vi "inter cycle delay tester.vi"() -> ()   [LabVIEW 2021]
uses:
  <vilib>/Analysis/1siggen.llb/Ramp Pattern by Samples.vi
  <vilib>/Analysis/NI_AALBase.lvlib
panel:
  out "second subarray":bool[](array[boolean])
  out "unsigned 8bit integer":u8
  out "Waveform Graph":i16[][](graph)
  out "delayed data":i16[][](array[numeric])
  in  "delay":u8
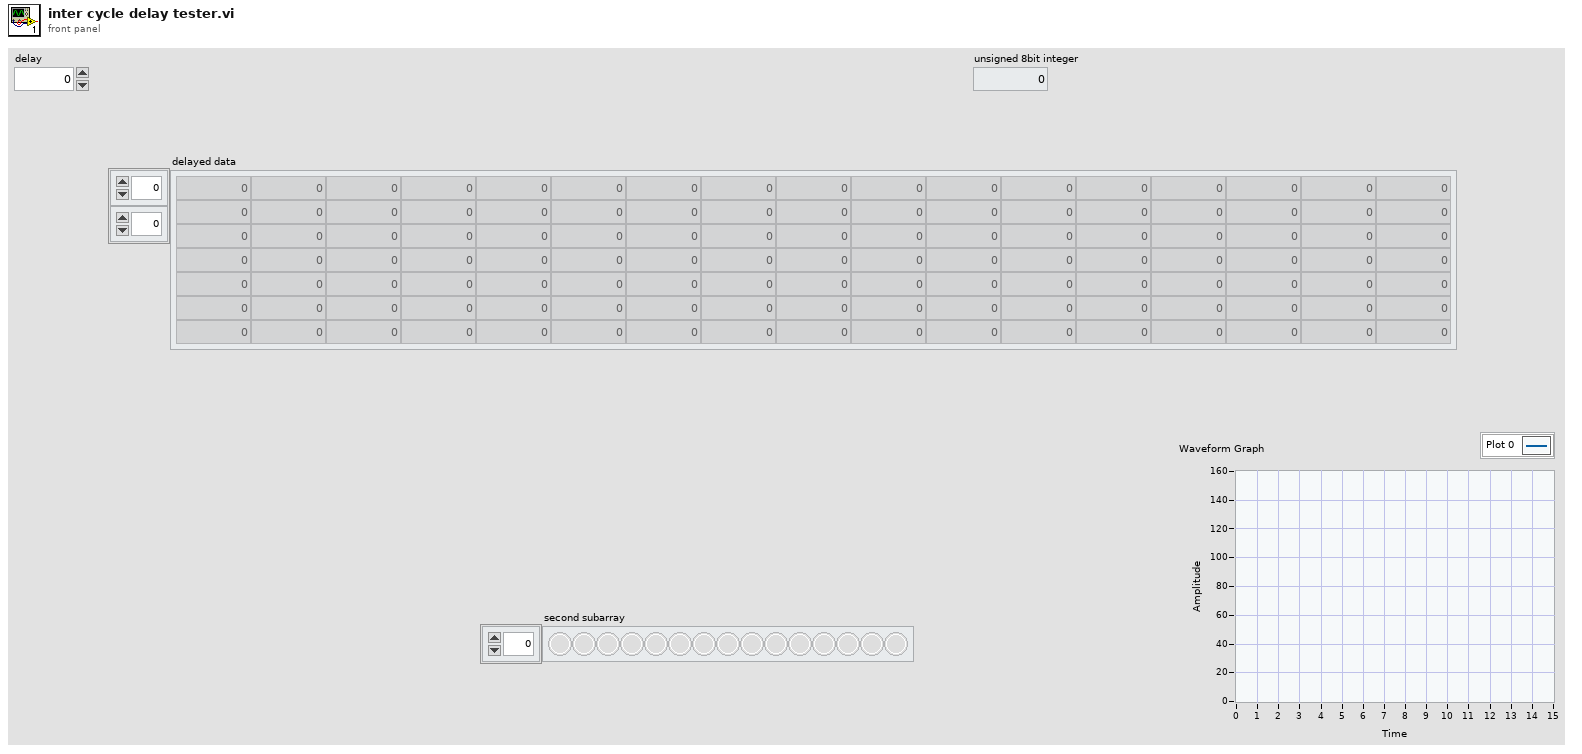
[diagram p1: front panel]
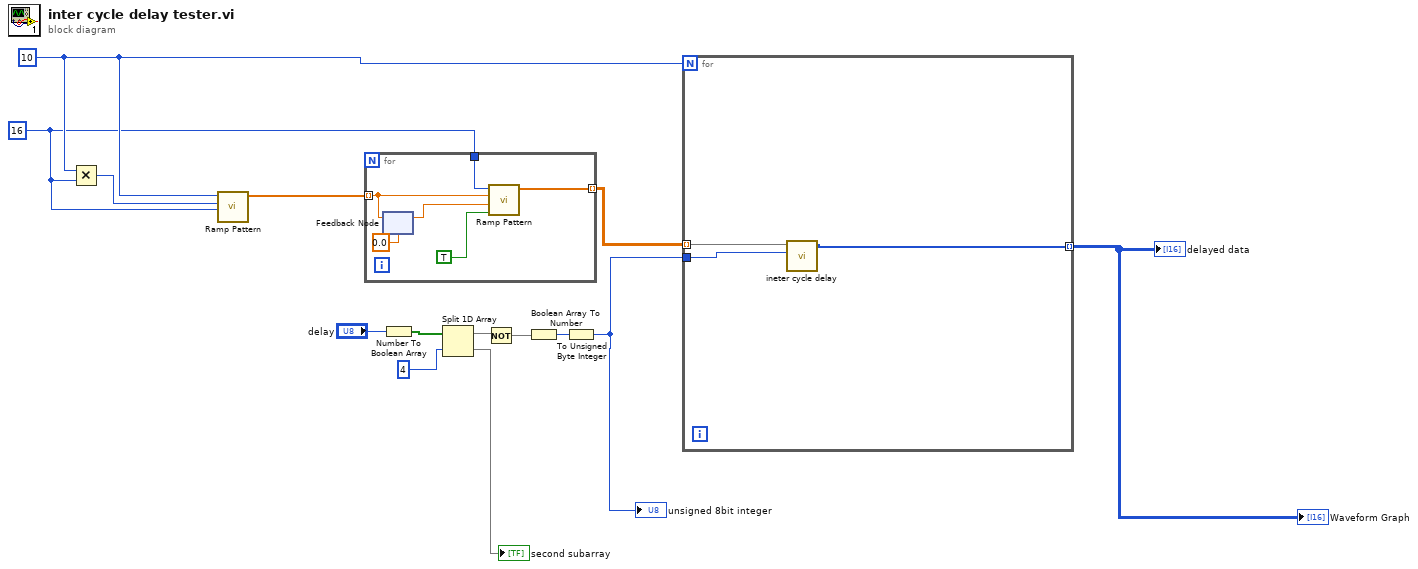
[diagram p0: block diagram]
diagram:
  w10 = 16 ("samples")
  w14 = 10
  n1 = Multiply(x=w14, y=w10) -> (x*y=w13:i32)
  n2 = call-poly <vilib>:"Ramp Pattern.vi"("start"=w10, "end"=w13, "samples"=w14) -> ("Ramp Pattern"=w12:dbl[])  [unwired: 7 in, 1 out]
  n3 = for {
    tunnel: w10 -> [w20]
    tunnel: w12 -> [w19] mode=indexing
    tunnel: [w16] -> w11 mode=indexing
    n4 = feedback-in #1(w19) -> ()
    n5 = feedback #1(0.0) -> (w18:dbl)
    n6 = call-poly <vilib>:"Ramp Pattern.vi"("exclude end?"=TRUE, "start"=w18, "end"=w19, "samples"=w20) -> ("Ramp Pattern"=w16:dbl[])  [unwired: 6 in, 1 out]
  }
  n7 = Number To Boolean Array(number="delay") -> (Boolean array=w7:bool[])
  n8 = Split 1D Array(array=w7, index=4) -> (first subarray=w5:bool[], second subarray=→"second subarray":bool[])
  n9 = Not(x=w5) -> (.not. x?=w4:bool[])
  n10 = Boolean Array To Number(Boolean array=w4) -> (number=w3:u32)
  n11 = To Unsigned Byte Integer(number=w3) -> (unsigned 8bit integer=w2:u8)
  "unsigned 8bit integer" <- w2
  n12 = for {
    N: w14 -> [_]
    tunnel: w2 -> [w23]
    tunnel: w11 -> [w22] mode=indexing
    tunnel: [w21] -> w9 mode=indexing
    n13 = call "ineter cycle delay.vi"("delay"=w23, "array in"=w22) -> ("delayed data"=w21:i16[])  [unwired: 9 in]
  }
  "delayed data" <- w9
  "Waveform Graph" <- w9
